vi "Read_Write_Test_Parameters.vi"(7 "Task":enum16{"Save", "Read", "Clear"}(ring)=enum."Read", 9 "Instrument Name":string(combo), 11 "Settings":T1={"Name of test"="", "Date"=timestamp(0 s since 1904-01-01), "Location"="", "Template"="", "Soundcard"="", "resolution"=32, "Sampling rate"=48000, "Ch1 Gain "=25.0, "Ch2 Gain"=10.0, "Sample time (s)"=0.3, "Pre-trigger (s)"=0.01, "Hammer Threshold"=10.0, "Positions"=12, "Taps/Position"=5, "Set Names"="", "Freq resolution"=10.0, "Hammer cutoff"=0.0, "Mic cutoff"=0.0, "Double bounce "=0.0, "Hammer Cal"=10.0, "dB Offset"=0.0, "Accel Cal"=10.0, "Vibrometer Cal"=0.0, "Mic Cal"=0.0, "Output"=2, "Voltage Cal"=1.0, "Vibrometer Port"="ASRL27::INSTR", "Range"=4, "High Pass"=2, "Bandwidth"=4, "X Range"=[], "Y Range"=[], "dB Spread"=0.0, "Trigger"=0, "Ch_1"=25, "Ch_2"=25, "flip?"=FALSE, "60Hz"=FALSE, "Time offset"=0.0, "Piezo Cal"=1.0, "Default Notes"=""} {"Ch_2" min=1 step=1; "Ch_1" min=1 max=100 step=1; "Trigger" items=["Hammer (force)", "Self-tap", "Spacebar"]; "Bandwidth" items=["1 kHz"=1, "5 kHz"=5, "10 kHz"=10, "25 kHz"=25, "50 kHz"=50, "100 kHz"=100]; "High Pass" items=["Off", "13 Hz", "104 Hz"]; "Range" items=["10 mm/s"=1, "20 mm/s"=2, "50 mm/s"=5, "100 mm/s"=10, "200 mm/s"=20, "500 mm/s"=50, "1 m/s"=100, "2 m/s"=200]; "Output" items=["Accelerometer", "Speed (from acceleration)", "Microphone", "Vibrometer", "Piezo"]; "Voltage Cal" format="%#_13g"; "Ch2 Gain" format="%#_13g"; "Ch1 Gain" format="%#_13g"; "Double bounce" min=0.0; "Mic cutoff" min=0.0 format="%#_4g"; "Hammer cutoff" min=0.0 format="%#_4g"; "Freq resolution" min=0.0; "Pre-trigger (s)" format="%#_13g"; "Date" format="%<%H:%M\n%d/%m/%y>T"; "resolution" items=["16 bit"=16, "24 bit"=24, "32 bit"=32]; "Sampling rate" items=["22050 samp/s"=22050, "44100 samp/s"=44100, "48000 samp/s"=48000]}) -> (0 "Exists?":bool, 3 "Settings":T1={"Name of test"="", "Date"=timestamp(0 s since 1904-01-01), "Location"="", "Template"="", "Soundcard"="", "resolution"=32, "Sampling rate"=48000, "Ch1 Gain "=25.0, "Ch2 Gain"=10.0, "Sample time (s)"=0.3, "Pre-trigger (s)"=0.01, "Hammer Threshold"=10.0, "Positions"=12, "Taps/Position"=5, "Set Names"="", "Freq resolution"=10.0, "Hammer cutoff"=0.0, "Mic cutoff"=0.0, "Double bounce "=0.0, "Hammer Cal"=10.0, "dB Offset"=0.0, "Accel Cal"=10.0, "Vibrometer Cal"=0.0, "Mic Cal"=0.0, "Output"=2, "Voltage Cal"=1.0, "Vibrometer Port"="ASRL27::INSTR", "Range"=4, "High Pass"=2, "Bandwidth"=4, "X Range"=[], "Y Range"=[], "dB Spread"=0.0, "Trigger"=0, "Ch_1"=25, "Ch_2"=25, "flip?"=FALSE, "60Hz"=FALSE, "Time offset"=0.0, "Piezo Cal"=1.0, "Default Notes"=""} {"Ch_2" min=1 step=1; "Ch_1" min=1 max=100 step=1; "Trigger" items=["Hammer (force)", "Self-tap", "Spacebar"]; "Bandwidth" items=["1 kHz"=1, "5 kHz"=5, "10 kHz"=10, "25 kHz"=25, "50 kHz"=50, "100 kHz"=100]; "High Pass" items=["Off", "13 Hz", "104 Hz"]; "Range" items=["10 mm/s"=1, "20 mm/s"=2, "50 mm/s"=5, "100 mm/s"=10, "200 mm/s"=20, "500 mm/s"=50, "1 m/s"=100, "2 m/s"=200]; "Output" items=["Accelerometer", "Speed (from acceleration)", "Microphone", "Vibrometer", "Piezo"]; "Voltage Cal" format="%#_13g"; "Ch2 Gain" format="%#_13g"; "Ch1 Gain" format="%#_13g"; "Double bounce" min=0.0; "Mic cutoff" min=0.0 format="%#_4g"; "Hammer cutoff" min=0.0 format="%#_4g"; "Freq resolution" min=0.0; "Pre-trigger (s)" format="%#_13g"; "Date" format="%<%H:%M\n%d/%m/%y>T"; "resolution" items=["16 bit"=16, "24 bit"=24, "32 bit"=32]; "Sampling rate" items=["22050 samp/s"=22050, "44100 samp/s"=44100, "48000 samp/s"=48000]})   [LabVIEW 2022 SP3]
uses:
  PreferencesControl.ctl
  Mic/Mic_Global.vi
panel:
  out "Path to instrument":path
  out "error out":errorcluster
  in  "error in":errorcluster
  out "string":string
  # "Hz"
  # "dB"
  # "dB"
  # "sec"
  # "sec"
  # "mV/Pa"
  # "mV/m/s2"
  # "mV/mm/s"
  # "V/N"
  # "sec"
  # "sec"
  # "mV/N"
  # "a.u."
  # "a.u."
  # "sec"
  # "Hz"
  # "dB"
  # "dB"
  # "sec"
  # "sec"
  # "mV/Pa"
  # "mV/m/s2"
  # "mV/mm/s"
  # "V/N"
  # "sec"
  # "sec"
  # "mV/N"
  # "a.u."
  # "a.u."
  # "sec"
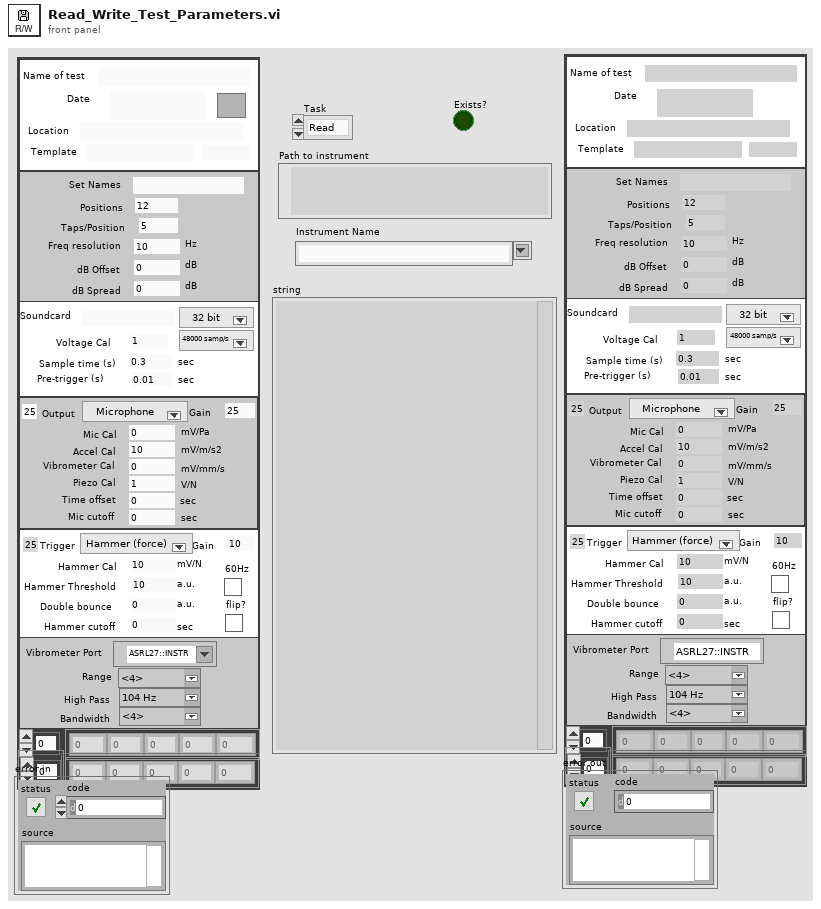
[diagram p1: front panel]
types:
  T1 = typedef "PreferencesControl.ctl" = cluster{"Name of test":string, "Date":timestamp, "Location":string, "Template":string, "Soundcard":string, "resolution":u16, "Sampling rate":u16, "Ch1 Gain ":dbl, "Ch2 Gain":dbl, "Sample time (s)":dbl, "Pre-trigger (s)":dbl, "Hammer Threshold":dbl, "Positions":i16, "Taps/Position":i16, "Set Names":string, "Freq resolution":dbl, "Hammer cutoff":dbl, "Mic cutoff":dbl, "Double bounce ":dbl, "Hammer Cal":dbl, "dB Offset":dbl, "Accel Cal":dbl, "Vibrometer Cal":dbl, "Mic Cal":dbl, "Output":u16, "Voltage Cal":dbl, "Vibrometer Port":refnum<visa-resource-name>, "Range":u16, "High Pass":u16, "Bandwidth":u16, "X Range":cluster{"Minimum":dbl, "Maximum":dbl, "Increment":dbl, "Minor Increment":dbl, "Start":dbl}[], "Y Range":cluster{"Minimum":dbl, "Maximum":dbl, "Increment":dbl, "Minor Increment":dbl, "Start":dbl}[], "dB Spread":dbl, "Trigger":u16, "Ch_1":u8, "Ch_2":u8, "flip?":bool, "60Hz":bool, "Time offset":dbl, "Piezo Cal":dbl, "Default Notes":string}
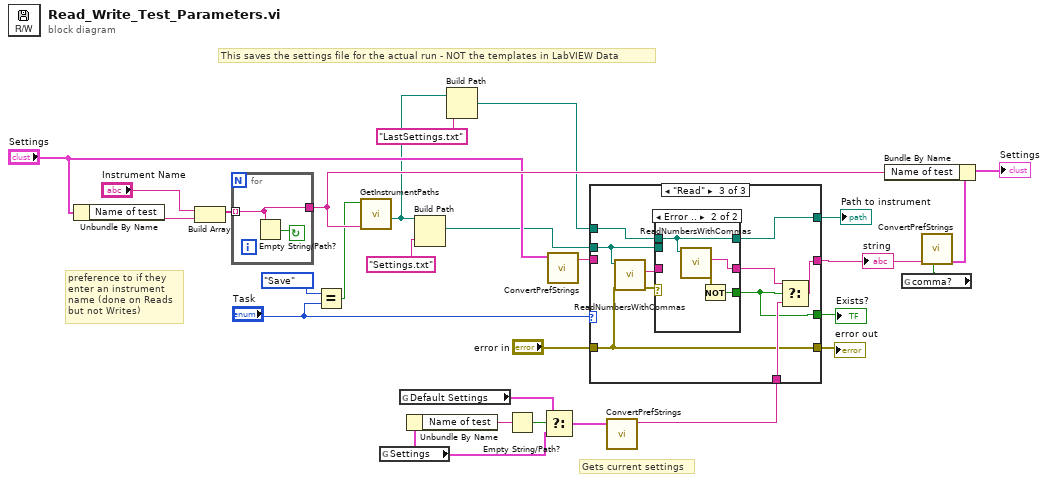
[diagram p0: block diagram]
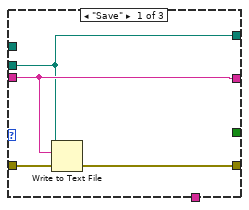
[diagram p2: hidden frame]
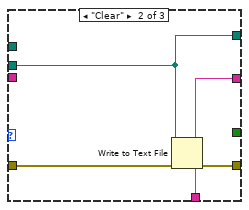
[diagram p3: hidden frame]
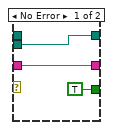
[diagram p4: hidden frame]
diagram:
  # "This saves the settings file for the actual run - NOT the templates in LabVIEW Data"
  # "preference to if they\nenter an instrument \nname (done on Reads\nbut not Writes)"
  # "Gets current settings"
  n1 = Unbundle By Name("Settings") -> ("Name of test"=w25:string)
  n2 = Build Array("Instrument Name", w25) -> (w24:string[])
  n3 = for {
    tunnel: w24 -> [w30] mode=indexing
    tunnel: [w30] -> w23
    stop <- w29 continue-if-true
    n4 = Empty String/Path?(string/path=w30) -> (empty?=w29:bool)
  }
  n5 = Equal?(x=enum16{"Save", "Read", "Clear"}."Save", y="Task") -> (x = y?=w6:bool)
  n6 = call "GetInstrumentPaths.vi"("Instrument"=w23, "Build?"=w6) -> ("Path To Test Folder"=w5:path)  [unwired: 5 in, 4 out]
  n7 = global read "Mic_Global.vi" "Settings"() -> (w10:T1)
  n8 = global read "Mic_Global.vi" "Default Settings"() -> (w11:T1)
  n9 = Unbundle By Name(w10) -> ("Name of test"=w13:string)
  n10 = Build Path(base path=w5, name or relative path="Settings.txt") -> (appended path=w17:path)
  n11 = Build Path(base path=w5, name or relative path="LastSettings.txt") -> (appended path=w3:path)
  n12 = Empty String/Path?(string/path=w13) -> (empty?=w12:bool)
  n13 = Select(t=w11, s=w12, f=w10) -> (s? t:f=w9:T1)
  n14 = call "ConvertPrefStrings.vi"("Settings"="Settings") -> ("String Out"=w21:string)  [unwired: 9 in, 1 out]
  n15 = call "ConvertPrefStrings.vi"("Settings"=w9) -> ("String Out"=w18:string)  [unwired: 9 in, 1 out]
  n16 = case shown="\"Read\"" "Task" {
    tunnel: [w34 w38 w48] -> w15
    tunnel: "error in" -> [w33 w37 w39]
    tunnel: [w32 w36 w39] -> w19
    tunnel: w17 -> [w31 w35 w40]
    tunnel: w21 -> [w34 _ _]
    tunnel: w18 -> [_ w38 w47]
    tunnel: [_ _ w44] -> w27
    tunnel: w3 -> [_ _ w45]
    tunnel: [w31 w35 w43] -> w2
    frame "Save" {
      n17 = Write to Text File(file (use dialog)=w31, text=w34, error in=w33) -> (error out=w32:errorcluster)  [unwired: 1 in, 2 out]
    }
    frame "Clear" {
      n18 = Write to Text File(file (use dialog)=w35, text=w38, error in=w37) -> (error out=w36:errorcluster)  [unwired: 1 in, 2 out]
    }
    frame "Read" {
      n19 = call "ReadNumbersWithCommas.vi"("error in"=w39, "file (use dialog)"=w40) -> ("error out"=w42:errorcluster, "text"=w41:string)  [unwired: 6 in, 2 out]
      n20 = case shown="Error .." w42 {
        tunnel: [w51 w53] -> w46
        tunnel: w41 -> [w51 _]
        tunnel: w45 -> [_ w54]
        tunnel: [TRUE w55] -> w44
        tunnel: [w49 w54] -> w43
        tunnel: w40 -> [w49 _]
        frame No Error {
        }
        frame Error {
          n21 = call "ReadNumbersWithCommas.vi"("file (use dialog)"=w54) -> ("error out"=w52:errorcluster, "text"=w53:string)  [unwired: 7 in, 2 out]
          n22 = Not(x=w52) -> (.not. x?=w55:bool)
        }
      }
      n23 = Select(t=w46, s=w44, f=w47) -> (s? t:f=w48:string)
    }
  }
  "string" <- w15
  "error out" <- w19
  "Path to instrument" <- w2
  "Exists?" <- w27
  n24 = global read "Mic_Global.vi" "comma?"() -> (w1:bool)
  n25 = call "ConvertPrefStrings.vi"("Comma?"=w1, "String In"=w15) -> ("Settings"=w20:T1)  [unwired: 8 in, 1 out]
  n26 = Bundle By Name(cluster=w20, "Name of test"=w23) -> (→"Settings":T1)
